vi "DestroySelfReference.vi"(8 "error in (no error)":errorcluster, 11 "SMO":refnum<class "SMO.lvclass">) -> (0 "error out":errorcluster, 3 "SMO out":refnum<class "SMO.lvclass">)   [LabVIEW 2021, in "smo.lvlib" / "SMO.lvclass"]
uses:
  SMO.lvclass
  SMO.lvclass/SMO.ctl
  Support/Attribute.Owner/Attribute.Owner.lvclass/Attribute.Owner.ctl
  Private/GetVariant(Attr).vi
  Support/Attribute.Owner/Attribute.Owner.lvclass
panel:
  # "For instructions on how to use the JKI State Machine Objects, examples and video tutorials, visit:\nhttp://jki.net/state-machine-objects/\n\nJKI State Machine Objects™\nhttp://jki.net/state-machine-objects/\nCopyright (C) 2005-2015, JKI <info@jki.net>\nALL RIGHTS RESERVED"
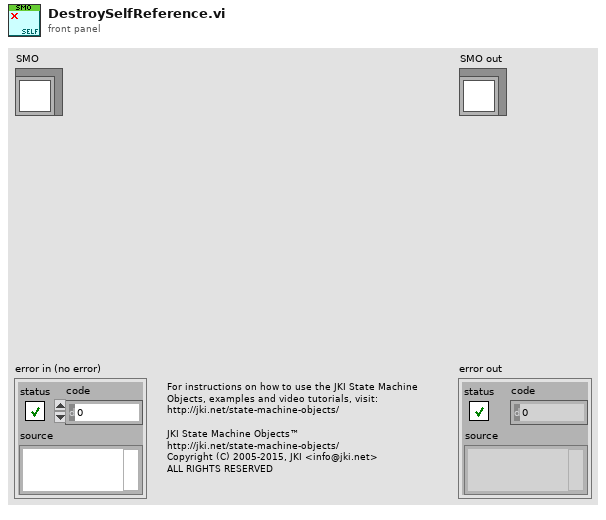
[diagram p1: front panel]
types:
  T1 = typedef "smo.lvlib/SMO.lvclass/PrivateData--Ref.ctl" = refnum<data-value>
  T2 = typedef "smo.lvlib/SMO.lvclass/PrivateData--Cluster.ctl" = cluster{"Parent Call":T3, "Registered Processes":T4[], "Sync Notifier":refnum<notifier>, "Process Error Notifier":refnum<notifier>, "Protected Events":T5, "Public Events":T6, "SMO State":T7, "[Attributes]":variant, "Launcher Close":refnum<notifier>, "Caller Watchdog":refnum<queue>, "Accessibility":T8, "NbStaticDependencies":u32}
  T3 = typedef "smo.lvlib/SMO.lvclass/Parent Call--Enum.ctl" = enum16{"Allows parent to run", "Does not request parent to run"}
  T4 = typedef "smo.lvlib/SMO.lvclass/RegisteredProcessData--Cluster.ctl" = cluster{"Name":string, "Static VI Ref":refnum<vi>, "Running":bool, "NotifierRef":u32}
  T5 = typedef "smo.lvlib/SMO.lvclass/Protected Events.ctl" = cluster{"StopProcesses":refnum<user-event>, "AbortProcesses":refnum<user-event>, "Config Changed":refnum<user-event>, "Dependency":refnum<user-event>}
  T6 = typedef "smo.lvlib/SMO.lvclass/Public Events.ctl" = cluster{"Error":refnum<user-event>, "State":refnum<user-event>, "Reserve State":refnum<user-event>}
  T7 = typedef "smo.lvlib/SMO.lvclass/SMOState --Enum.ctl" = enum16{"unknown", "Created", "Started", "Stopped"}
  T8 = typedef "smo.lvlib/SMO.lvclass/Accessibility--Cluster.ctl" = cluster{"Lock Key":string, "Reserve State":T9}
  T9 = typedef "smo.lvlib/SMO.lvclass/Reserve State--Enum.ctl" = enum16{"Unreserved", "Reserved", "Self-locked"}
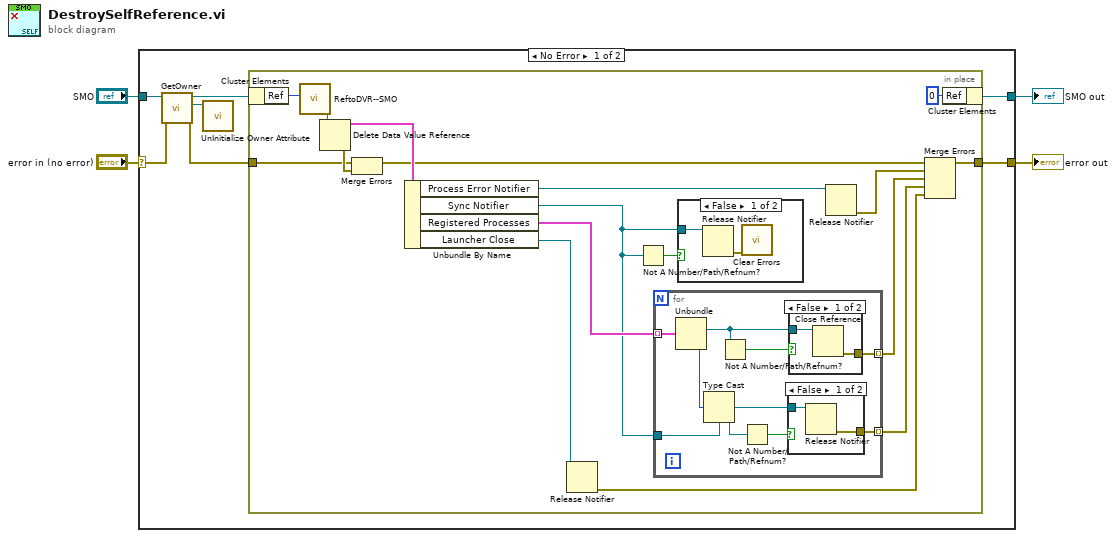
[diagram p0: block diagram]
diagram:
  n1 = case shown="No Error" "error in (no error)" {
    selector: "error in (no error)" -> [w7 w45]
    tunnel: [w11 w45] -> w3
    tunnel: [w10 w44] -> w1
    tunnel: "SMO" -> [w9 w44]
    frame No Error {
      n2 = call "GetOwner.vi"("error in (no error)"=w7, "SMO in"=w9) -> ("error out"=w6:errorcluster, "Owner"=w5:refnum<class "Attribute.Owner.lvclass">, "SMO out"=w8:refnum<class "SMO.lvclass">)  [unwired: 6 in, 1 out]
      n3 = call "UnInitialize Owner Attribute.vi"("Attribute.Owner"=w5) -> ()  [unwired: 11 in]
      n4 = in-place {
        in-place-border: w6 -> [w21]
        in-place-border: [w28] -> w11
        n5 = in-place-cluster #1(w8) -> ("Ref"=w18:u32)
        n6 = call "ReftoDVR--SMO.vi"("Ref"=w18) -> ("Ref"=w17:T1)  [unwired: 10 in]
        n7 = Delete Data Value Reference(data value reference=w17) -> (data value=w25:T2, error out=w22:errorcluster)  [unwired: 1 in]
        n8 = Merge Errors(w21, w22) -> (w20:errorcluster)
        n9 = Unbundle By Name(w25) -> ("Process Error Notifier"=w26:refnum<notifier>, "Sync Notifier"=w13:refnum<notifier>, "Registered Processes"=w27:T4[], "Launcher Close"=w16:refnum<notifier>)
        n10 = Release Notifier(notifier=w16) -> (error out=w14:errorcluster)  [unwired: 2 in, 2 out]
        n11 = Not A Number/Path/Refnum?(number/path/refnum=w13) -> (NaN/Path/Refnum?=w12:bool)
        n12 = for {
          tunnel: w27 -> [w38] mode=indexing
          tunnel: [w36] -> w23 mode=indexing
          tunnel: w13 -> [w34]
          tunnel: [w31] -> w15 mode=indexing
          n13 = Unbundle(w38) -> ("Static VI Ref"=w37:refnum<vi>, "NotifierRef"=w35:u32)  [unwired: 2 out]
          n14 = Type Cast(type=w34, x=w35) -> (*(type *) &x=w33:refnum<notifier>)
          n15 = Not A Number/Path/Refnum?(number/path/refnum=w37) -> (NaN/Path/Refnum?=w39:bool)
          n16 = Not A Number/Path/Refnum?(number/path/refnum=w33) -> (NaN/Path/Refnum?=w32:bool)
          n17 = case shown="False" w32 {
            tunnel: w33 -> [w41 _]
            tunnel: [w40 _] -> w31
            frame False {
              n18 = Release Notifier(notifier=w41) -> (error out=w40:errorcluster)  [unwired: 2 in, 2 out]
            }
            frame True {
            }
          }
          n19 = case shown="False" w39 {
            tunnel: w37 -> [w43 _]
            tunnel: [w42 _] -> w36
            frame False {
              n20 = Close Reference(reference=w43) -> (error out=w42:errorcluster)  [unwired: 1 in]
            }
            frame True {
            }
          }
        }
        n21 = case shown="False" w12 {
          tunnel: w13 -> [w29 _]
          frame False {
            n22 = Release Notifier(notifier=w29) -> (error out=w30:errorcluster)  [unwired: 2 in, 2 out]
            n23 = call <vilib>:"Clear Errors.vi"("error in (no error)"=w30) -> ()  [unwired: 5 in, 2 out]
          }
          frame True {
          }
        }
        n24 = Release Notifier(notifier=w26) -> (error out=w24:errorcluster)  [unwired: 2 in, 2 out]
        n25 = Merge Errors(w20, w24, w23, w15, w14) -> (w28:errorcluster)
        n26 = in-place-cluster #1("Ref"=u32 0) -> (w10:refnum<class "SMO.lvclass">)
      }
    }
    frame Error {
    }
  }
  "error out" <- w3
  "SMO out" <- w1
